vi "LEFT Motion Profile Traj Points Array.vi"(10 "Read = false, Write = true":bool, 11 "traj. points array in":dbl[][](array[numeric])) -> (3 "traj. points array out":dbl[][](array[numeric]))   [LabVIEW 2018]
uses:
  <vilib>/Rock Robotics/Network Tables/NT Read Numeric Array.vi
  <vilib>/Rock Robotics/Network Tables/NT Write Numeric Array.vi
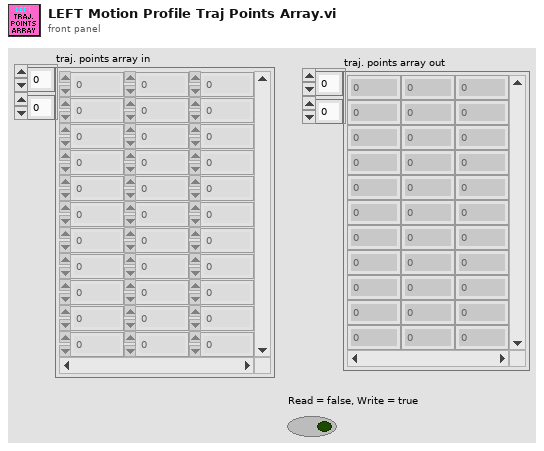
[diagram p1: front panel]
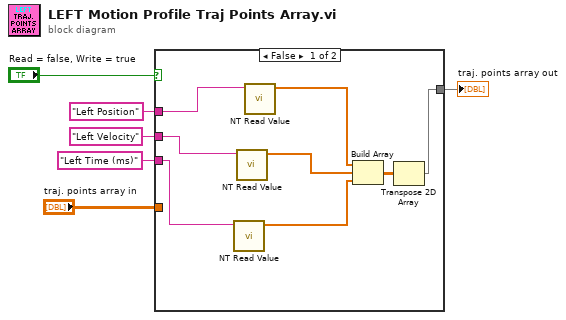
[diagram p0: block diagram]
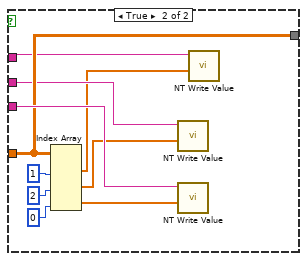
[diagram p2: hidden frame]
diagram:
  n1 = case shown="False" "Read = false, Write = true" {
    tunnel: "traj. points array in" -> [_ w19]
    tunnel: "Left Position" ("Name") -> [w13 w15]
    tunnel: "Left Velocity" ("Name") -> [w14 w17]
    tunnel: "Left Time (ms)" ("Name") -> [w12 w20]
    tunnel: [w9 w19] -> w1
    frame False {
      n2 = call-poly <vilib>:"NT Read Value.vi"("Name"=w12) -> ("Numeric Array"=w11:dbl[])  [unwired: 9 in, 1 out]
      n3 = call-poly <vilib>:"NT Read Value.vi"("Name"=w14) -> ("Numeric Array"=w7:dbl[])  [unwired: 9 in, 1 out]
      n4 = call-poly <vilib>:"NT Read Value.vi"("Name"=w13) -> ("Numeric Array"=w8:dbl[])  [unwired: 9 in, 1 out]
      n5 = Build Array(w8, w7, w11) -> (w10:dbl[][])
      n6 = Transpose 2D Array(2D array=w10) -> (transposed array=w9:dbl[][])
    }
    frame True {
      n7 = Index Array(array=w19, index (col) #1=1 ("disabled index (col)"), index (col) #2=2 ("index (col)"), index (col) #3=0 ("index (col)")) -> (element #1=w16:dbl[], element #2=w18:dbl[], element #3=w24:dbl[])  [unwired: 3 in]
      n8 = call-poly <vilib>:"NT Write Value.vi"("Numeric Array"=w18, "Name"=w17) -> ()  [unwired: 9 in, 1 out]
      n9 = call-poly <vilib>:"NT Write Value.vi"("Numeric Array"=w24, "Name"=w20) -> ()  [unwired: 9 in, 1 out]
      n10 = call-poly <vilib>:"NT Write Value.vi"("Numeric Array"=w16, "Name"=w15) -> ()  [unwired: 9 in, 1 out]
    }
  }
  "traj. points array out" <- w1
